vi "Create_population.vi"(11 "lambda":dbl=0.1 format="%#_13g") -> (3 "People":T1[](array[typedef]))   [LabVIEW 2014]
doc: "Przyjmuje lambda (liczbę klientów na jednostkę czasu). Zwraca tablicę tysiąca ludzi."
uses:
  Client.ctl
  LukiBrary.lvlib
panel:
  out "Wartość oczekiwana (1/lambda)?":dbl
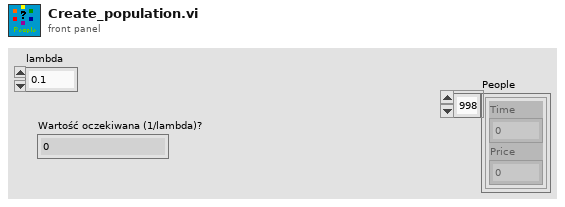
[diagram p1: front panel]
types:
  T1 = typedef "LukiBrary.lvlib/Client.ctl" = cluster{"Time":i32, "Price":i32}
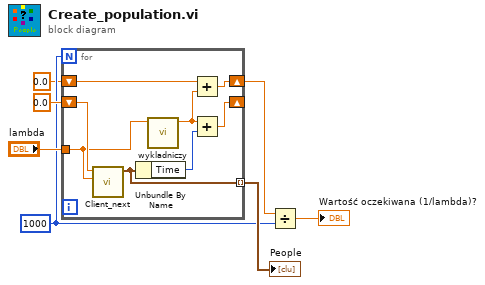
[diagram p0: block diagram]
diagram:
  w4 = 1000
  n1 = for {
    N: w4 -> [_]
    shift-right: [w14] -> _
    shift-left: 0.0 -> [w13]
    tunnel: "lambda" -> [w8]
    tunnel: [w12] -> w5 mode=indexing
    shift-right: [w9] -> w1
    shift-left: 0.0 -> [w10]
    n2 = call "Client_next.vi"("lambda"=w8, "Time of previous"=w13) -> ("Client"=w12:T1)  [unwired: 9 in]
    n3 = Unbundle By Name(w12) -> ("Time"=w15:i32)
    n4 = call "wykladniczy.vi"("lambda"=w8) -> ("X~wykładniczy"=w11:dbl)  [unwired: 10 in]
    n5 = Add(x=w10, y=w11) -> (x+y=w9:dbl)
    n6 = Add(x=w11, y=w15) -> (x+y=w14:dbl)
  }
  "People" <- w5
  n7 = Divide(x=w1, y=w4) -> (x/y=→"Wartość oczekiwana (1/lambda)?":dbl)
